vi "RB2 find all the dots.vi"(0 "Image In":T2, 1 "error in":errorcluster) -> (2 "Image Out":T2, 3 "All Found?":bool, 4 "Dot Array":T1(array[cluster]), 5 "error out":errorcluster)   [LabVIEW 2012]
doc: "This VI call the the \"find dot\" subroutines and outputs the first dots found for each color and a boolean positive when all the dots have been found."
uses:
  <vilib>/vision/Image Controls.llb/IMAQ Image.ctl
panel:
  out "Num of\nGreen  Dots":i32
  out "Green Dot\nLocation":T3(array[cluster])
  out "Blue Dot\nLocation":T3(array[cluster])
  out "Num of\nBlue Dots":i32
  out "Num of\nRed Dots":i32
  out "Red Dot\nLocation":T3(array[cluster])
  out "Black dot\nLocation":T3(array[cluster])
  out "Num Black\ndots":i32
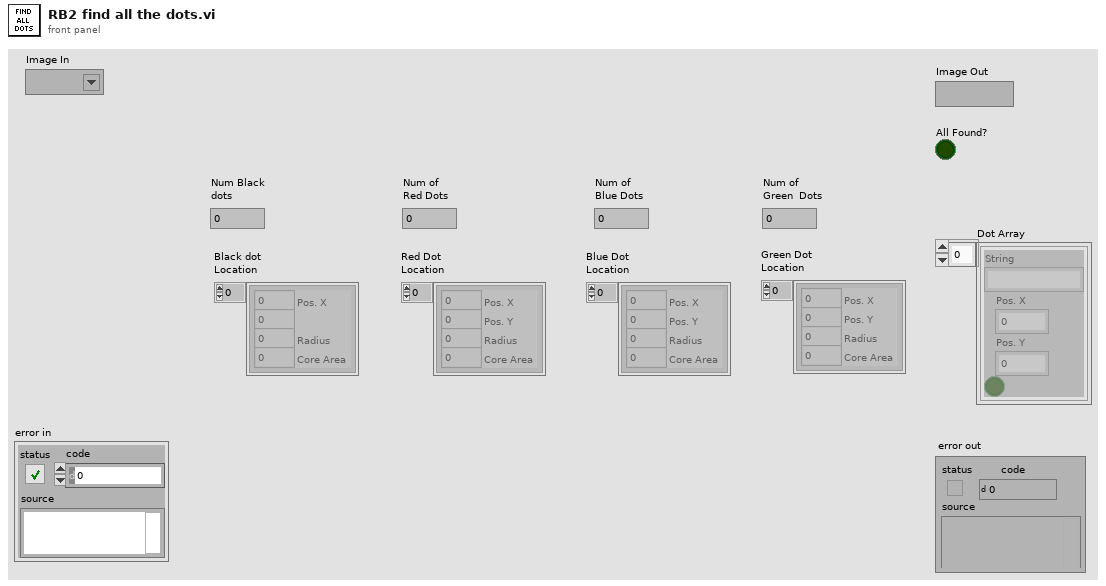
[diagram p1: front panel]
types:
  T1 = cluster{"String":string, "Pos. X":i32, "Pos. Y":i32, bool}[]
  T2 = typedef "IMAQ Image.ctl" = refnum<image>
  T3 = cluster{"Pos. X":i32, "Pos. Y":i32, "Radius":i32, "Core Area":i32}[]
  T4 = cluster{"String":string, "Pos. X":i32, "Pos. Y":i32, bool}
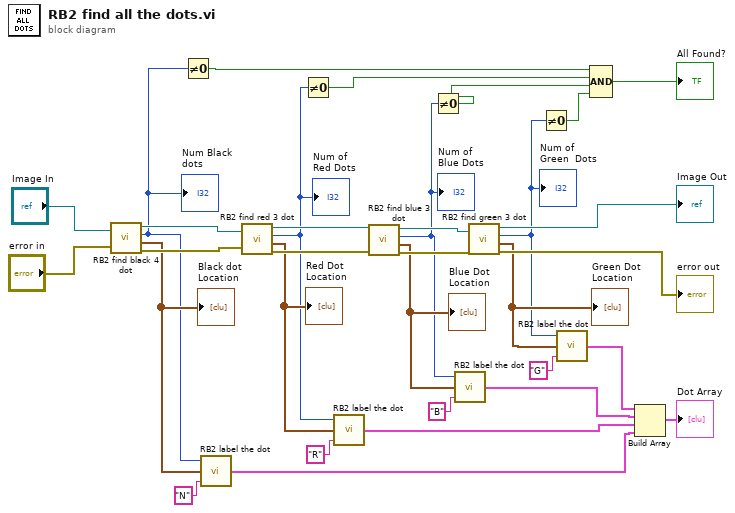
[diagram p0: block diagram]
diagram:
  n1 = call "RB2 find black 4 dot.vi"("Image In"="Image In", "error in"="error in") -> ("Image Out"=w31:T2, "Num Black\ndots"=w16:i32, "Black dot\nLocation"=w17:T3, "error out"=w32:errorcluster)
  "Num Black\ndots" <- w16
  "Black dot\nLocation" <- w17
  n2 = Not Equal To 0?(x=w16) -> (x != 0?=w22:bool)
  n3 = call "RB2 label the dot.vi"("Dot Name"="N", "Dot Location"=w17, "Num Dots"=w16) -> ("Dot Data"=w2:T4)
  n4 = call "RB2 find red 3 dot.vi"("Image In"=w31, "error in"=w32) -> ("Image Out"=w29:T2, "Num of\nRed Dots"=w12:i32, "Red Dot\nLocation"=w13:T3, "error out"=w30:errorcluster)
  "Red Dot\nLocation" <- w13
  "Num of\nRed Dots" <- w12
  n5 = Not Equal To 0?(x=w12) -> (x != 0?=w21:bool)
  n6 = call "RB2 label the dot.vi"("Dot Name"="R", "Dot Location"=w13, "Num Dots"=w12) -> ("Dot Data"=w3:T4)
  n7 = call "RB2 find blue 3 dot.vi"("Image In"=w29, "error in"=w30) -> ("Image Out"=w27:T2, "Num of\nBlue Dots"=w9:i32, "Blue Dot\nLocation"=w10:T3, "error out"=w28:errorcluster)
  "Num of\nBlue Dots" <- w9
  "Blue Dot\nLocation" <- w10
  n8 = Not Equal To 0?(x=w9) -> (x != 0?=w20:bool)
  n9 = call "RB2 label the dot.vi"("Dot Name"="B", "Dot Location"=w10, "Num Dots"=w9) -> ("Dot Data"=w4:T4)
  n10 = call "RB2 find green 3 dot.vi"("Image In"=w27, "error in"=w28) -> ("Image Out"=→"Image Out":T2, "Num of\nGreen  Dots"=w6:i32, "Green Dot\nLocation"=w7:T3, "error out"=→"error out":errorcluster)
  "Green Dot\nLocation" <- w7
  "Num of\nGreen  Dots" <- w6
  n11 = Not Equal To 0?(x=w6) -> (x != 0?=w19:bool)
  n12 = call "RB2 label the dot.vi"("Dot Name"="G", "Dot Location"=w7, "Num Dots"=w6) -> ("Dot Data"=w5:T4)
  n13 = Compound Arithmetic op=AND(w22, w21, w20, w19) -> (→"All Found?":bool)
  n14 = Build Array(w5, w4, w3, w2) -> (→"Dot Array":T1)
